vi "WriteCalcQ.vi"(8 "error in (no error)":errorcluster caption="entrée d'erreur (pas d'erreur)", 9 "CurrCrvPointInd":i32, 10 "DataIn":dbl[](array[numeric]), 11 "Interface en entrée":refnum<class "Interface.lvclass"> caption="DNL_LabVIEW Object in") -> (0 "error out":errorcluster caption="sortie d'erreur", 3 "Interface en sortie":refnum<class "Interface.lvclass"> caption="DNL_LabVIEW Object out")   [LabVIEW 2019, in "Interface.lvclass"]
uses:
  Interface.lvclass
panel:
  in  "CrvIndex":i32
  in  "CalcNameInd":i32[](array[numeric])
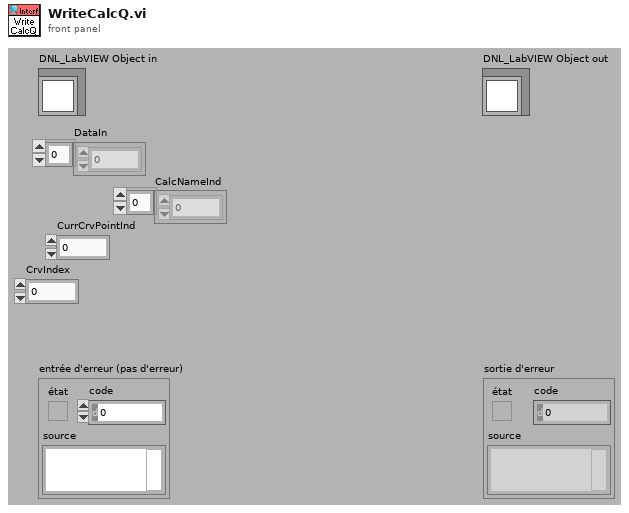
[diagram p1: front panel]
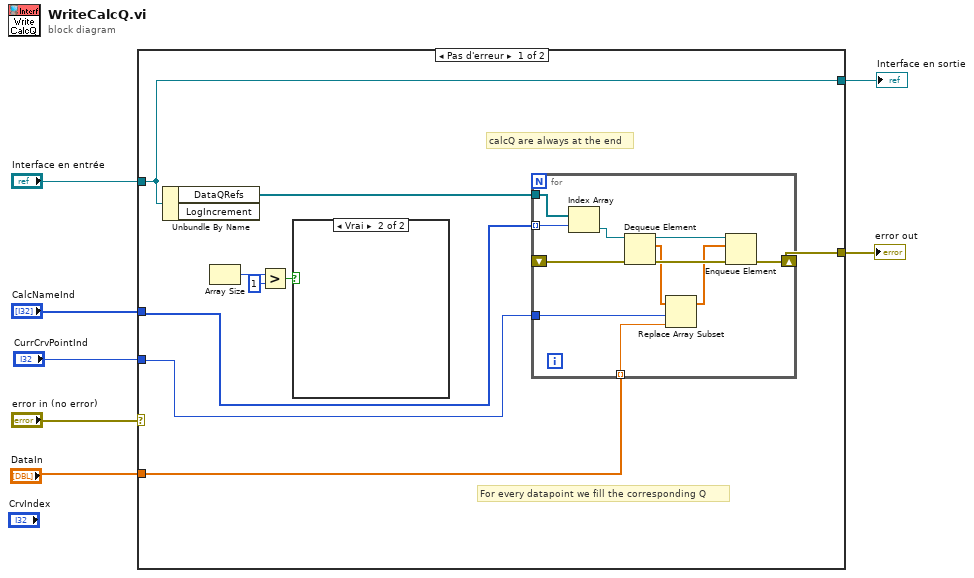
[diagram p0: block diagram]
diagram:
  n1 = case shown="Pas d'erreur" "error in (no error)" {
    selector: "error in (no error)" -> [_ w29]
    tunnel: [w16 w29] -> w6
    tunnel: [w15 w28] -> w4
    tunnel: "Interface en entrée" -> [w15 w28]
    tunnel: "DataIn" -> [w13 _]
    tunnel: "CurrCrvPointInd" -> [w8 _]
    tunnel: "CalcNameInd" -> [w9 _]
    frame No Error {
      # "For every datapoint we fill the corresponding Q"
      # "calcQ are always at the end"
      n2 = Unbundle By Name(w15) -> ("DataQRefs"=w14:refnum<queue>[])  [unwired: 1 out]
      n3 = Array Size() -> (size(s)=w12:i32)  [unwired: 1 in]
      n4 = Greater?(x=w12, y=1) -> (0:w10:bool)
      n5 = case shown="Vrai" w10 {
        frame False {
        }
        frame True {
        }
      }
      n6 = for {
        shift-right: [w26] -> w16
        shift-left: _ -> [w21]
        tunnel: w13 -> [w22] mode=indexing
        tunnel: w14 -> [w20]
        tunnel: w9 -> [w19] mode=indexing
        tunnel: w8 -> [w17]
        n7 = Index Array(array=w20, index=w19) -> (element=w18:refnum<queue>)
        n8 = Dequeue Element(queue=w18, error in (no error)=w21) -> (queue out=w27:refnum<queue>, element=w24:dbl[], error out=w25:errorcluster)  [unwired: 1 in, 1 out]
        n9 = Replace Array Subset(array=w24, new element=w22, index=w17) -> (w23:dbl[])
        n10 = Enqueue Element(queue=w27, element=w23, error in (no error)=w25) -> (error out=w26:errorcluster)  [unwired: 1 in, 2 out]
      }
    }
    frame Error {
    }
  }
  "error out" <- w6
  "Interface en sortie" <- w4
